vi "Winch v4.vi"() -> ()   [LabVIEW 2013]
uses:
  <vilib>/Rock Robotics/WPI/Joystick/WPI_JoystickGetSetRefNum.vi
  Robot Global Data.vi
  Globals/Useful Values.vi
  Globals/Homes.vi
  <vilib>/Utility/file.llb/Write To Spreadsheet File (DBL).vi
  <vilib>/addons/control/pid/pid.llb/PID (DBL).vi
  <vilib>/addons/control/pid/NI_PID_pid.lvlib
panel:
  in  "PID gains":T1={"proportional gain (Kc)"=2.75, "integral time (Ti, min)"=0.0, "derivative time (Td, min)"=0.0} {"derivative time (Td, min)" format="%.3f"; "integral time (Ti, min)" format="%.3f"; "proportional gain (Kc)" format="%.3f"}
  # "PULLBACK SPEED NEEDS\nTO BE NEGATIVE OR ELSE"
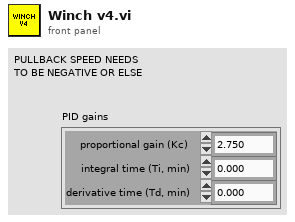
[diagram p1: front panel]
types:
  T1 = cluster{"proportional gain (Kc)":dbl, "integral time (Ti, min)":dbl, "derivative time (Td, min)":dbl}
  T2 = typedef "WPI_DigitalInputDevRef.ctl" = cluster{"DevStatus":errorcluster, "DIO Channel":T3, "Digital Module":T4}
  T3 = typedef "FPGA_DIOChannel.ctl" = enum8{"DIO 1", "DIO 2", "DIO 3", "DIO 4", "DIO 5", "DIO 6", "DIO 7", "DIO 8", "DIO 9", "DIO 10", "DIO 11", "DIO 12", "DIO 13", "DIO 14", "Invalid"}
  T4 = typedef "FPGA_TypedefDigitalModule.ctl" = enum16{"Digital Module 1", "Digital Module 2"}
  T5 = typedef "WPI_MotorControlDeviceRef.ctl" = cluster{"DeviceStatus":errorcluster, "Type":enum16{"PWM", "CAN"}, "PWM":cluster{"Digital Module":T4, "PWM Channel":T6, "DeadBand":T7}, "CAN":cluster{"Device Number":u8, "Control Mode":T8, "Semaphore":T9, "Max Vout":dbl}, "Invert":bool, "TransformRef":T10, "InvTransformRef":T10}
  T6 = typedef "FPGA_DIOPWMChannel.ctl" = enum8{"PWM 1", "PWM 2", "PWM 3", "PWM 4", "PWM 5", "PWM 6", "PWM 7", "PWM 8", "PWM 9", "PWM 10", "Invalid"}
  T7 = typedef "WPI_PWMDeadband.ctl" = cluster{"Name":string, "maxPositivePwm":i32, "minPositivePwm":i32, "centerPwm":i32, "maxNegativePwm":i32, "minNegativePwm":i32, "angularRange":u16}
  T8 = typedef "WPI_CANJaguar_ControlMode.ctl" = enum8{"Percent VBus", "Current", "Speed", "Position", "Voltage"}
  T9 = typedef "Semaphore RefNum" = refnum<k1>
  T10 = typedef "WPI_PWMTransform_ConPane.ctl" = refnum<vi>
  T11 = typedef "WPI_AnalogChannelDevRef.ctl" = cluster{"DevStatus":errorcluster, "Analog Module":T12, "Analog Channel":T13}
  T12 = typedef "FPGA_TypedefAnalogModule.ctl" = enum16{"Analog Module 1", "Analog Module 2"}
  T13 = typedef "FPGA_AIChannel.ctl" = enum8{"AI 1", "AI 2", "AI 3", "AI 4", "AI 5", "AI 6", "AI 7", "AI 8", "Invalid"}
  T14 = typedef "WPI_JoystickDevRef.ctl" = cluster{"Device":T15}
  T15 = typedef "WPI_JoystickDeviceEnum.ctl" = enum16{"USB 1", "USB 2", "USB 3", "USB 4", "Kinect 1", "Kinect 2"}
  T16 = typedef "WPI_DriverStationRobotMode2.ctl" = enum16{"Autonomous Disabled", "Autonomous Enabled", "Teleop Disabled", "Teleop Enabled", "Timeout", "Finish", "Test Disabled", "Test Enabled"}
  T17 = typedef "WPI_JoystickButtonState.ctl" = cluster{"Button 1":bool, "Button 2":bool, "Button 3":bool, "Button 4":bool, "Button 5":bool, "Button 6":bool, "Button 7":bool, "Button 8":bool, "Button 9":bool, "Button 10":bool, "Button 11":bool, "Button 12":bool}
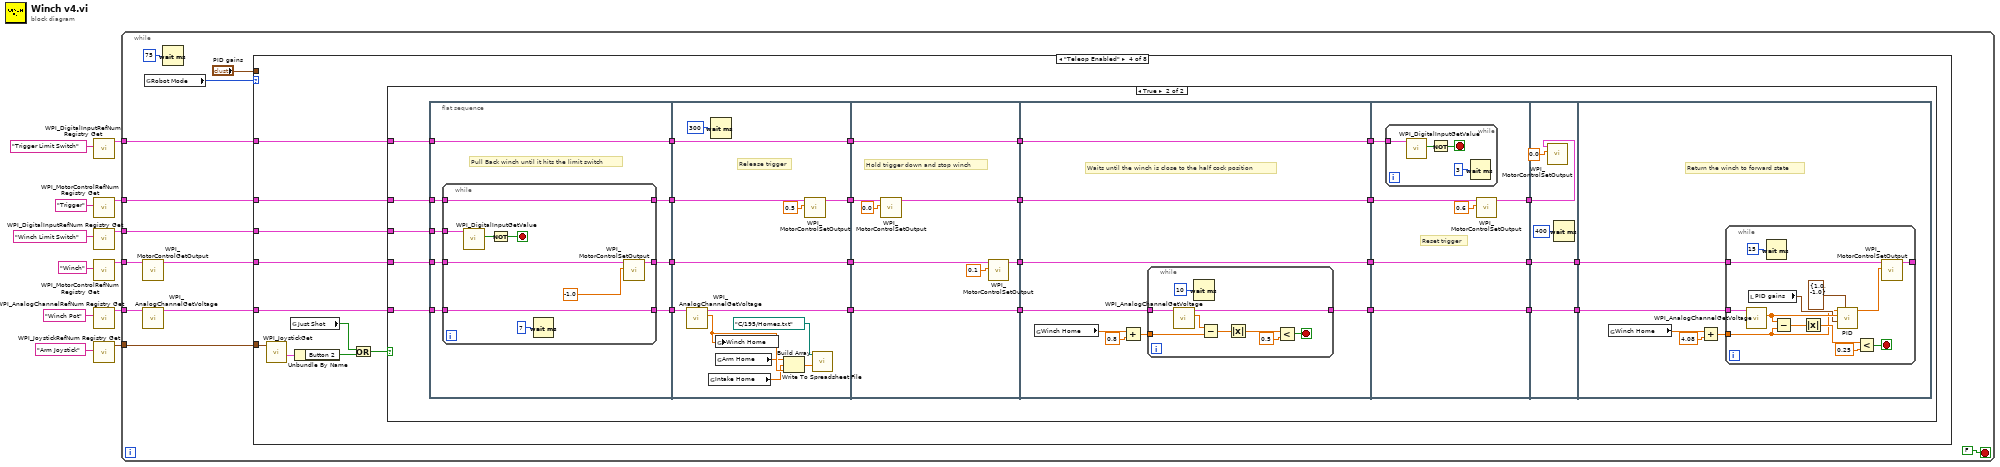
[diagram p0: block diagram]
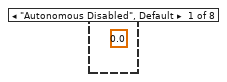
[diagram p2: hidden frame]
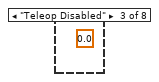
[diagram p4: hidden frame]
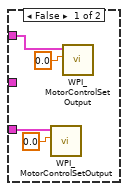
[diagram p5: hidden frame]
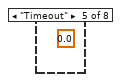
[diagram p6: hidden frame]
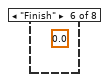
[diagram p7: hidden frame]
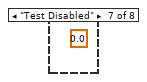
[diagram p8: hidden frame]
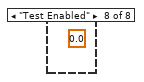
[diagram p9: hidden frame]
diagram:
  n1 = call <vilib>:"WPI_DigitalInputRefNum Registry Get.vi"("refnum name"="Trigger Limit Switch") -> ("DigitalInputDevRef"=w1:T2)  [unwired: 9 in, 1 out]
  n2 = call <vilib>:"WPI_MotorControlRefNum Registry Get.vi"("refnum name"="Trigger") -> ("MotorControlDevRef"=w3:T5)  [unwired: 9 in, 1 out]
  n3 = call <vilib>:"WPI_DigitalInputRefNum Registry Get.vi"("refnum name"="Winch Limit Switch") -> ("DigitalInputDevRef"=w6:T2)  [unwired: 9 in, 1 out]
  n4 = call <vilib>:"WPI_MotorControlRefNum Registry Get.vi"("refnum name"="Winch") -> ("MotorControlDevRef"=w9:T5)  [unwired: 9 in, 1 out]
  n5 = call <vilib>:"WPI_AnalogChannelRefNum Registry Get.vi"("refnum name"="Winch Pot") -> ("AIDeviceRef"=w12:T11)  [unwired: 9 in, 1 out]
  n6 = call <vilib>:"WPI_JoystickRefNum Registry Get.vi"("refnum name"="Arm Joystick") -> ("JoystickDevRef"=w7:T14)  [unwired: 9 in, 1 out]
  n7 = while {
    tunnel: w12 -> [w22]
    tunnel: w9 -> [w17]
    tunnel: w7 -> [w19]
    tunnel: w6 -> [w14]
    tunnel: w3 -> [w15]
    tunnel: w1 -> [w13]
    stop <- FALSE stop-if-true
    n8 = call <vilib>:"WPI_MotorControlGetOutput.vi"("MotorControlDevRef"=w17) -> ("MotorControlDevRef"=w16:T5)  [unwired: 8 in, 2 out]
    n9 = call <vilib>:"WPI_AnalogChannelGetVoltage.vi"("AIDeviceRef"=w22) -> ("AIDeviceRef"=w18:T11)  [unwired: 8 in, 2 out]
    n10 = global read "Robot Global Data.vi" "Robot Mode"() -> (w21:T16)
    n11 = Wait (ms)(milliseconds to wait=u32 75) -> ()  [unwired: 1 out]
    n12 = case shown="\"Teleop Enabled\"" w21 {
      tunnel: w16 -> [_ _ _ w31 _ _ _ _]
      tunnel: "PID gains" -> [_ _ _ _ _ _ _ _]
      tunnel: w19 -> [_ _ _ w34 _ _ _ _]
      tunnel: w14 -> [_ _ _ w32 _ _ _ _]
      tunnel: w18 -> [_ _ _ w30 _ _ _ _]
      tunnel: w15 -> [_ _ _ w26 _ _ _ _]
      tunnel: w13 -> [_ _ _ w25 _ _ _ _]
      frame "Autonomous Disabled", Default {
        (unwired) 0.0 ("Motor Output")
      }
      frame "Autonomous Enabled" {
      }
      frame "Teleop Disabled" {
        (unwired) 0.0 ("Motor Output")
      }
      frame "Teleop Enabled" {
        n13 = call <vilib>:"WPI_JoystickGet.vi"("JoystickDevRef"=w34) -> ("Buttons"=w33:T17)  [unwired: 4 in, 2 out]
        n14 = global read "Useful Values.vi" "Just Shot"() -> (w29:bool)
        n15 = Unbundle By Name(w33) -> ("Button 2"=w28:bool)
        n16 = Or(x=w29, y=w28) -> (x .or. y?=w27:bool)
        n17 = case shown="True" w27 {
          tunnel: w32 -> [_ w62]
          tunnel: w31 -> [w38 w64]
          tunnel: w30 -> [_ w63]
          tunnel: w26 -> [w35 w61]
          tunnel: w25 -> [_ w47]
          frame False {
            n18 = call <vilib>:"WPI_MotorControlSetOutput.vi"("Output"=0.0, "MotorControlDevRef"=w38) -> ()  [unwired: 7 in, 3 out]
            n19 = call <vilib>:"WPI_MotorControlSetOutput.vi"("Output"=0.0, "MotorControlDevRef"=w35) -> ()  [unwired: 7 in, 3 out]
          }
          frame True {
            n20 = flat-sequence {
              tunnel: w64 -> [w72]
              tunnel: w63 -> [w71]
              tunnel: w62 -> [w70]
              tunnel: w61 -> [w68]
              tunnel: [w69] -> w60
              tunnel: [w67] -> w57
              tunnel: [w66] -> w56
              tunnel: [w65] -> w48
              tunnel: w47 -> [w65]
              tunnel: w60 -> [w94]
              tunnel: [w91] -> w59
              tunnel: [w90] -> w58
              tunnel: w57 -> [w90]
              tunnel: w56 -> [w83]
              tunnel: [w82] -> w55
              tunnel: [w89] -> w49
              tunnel: w48 -> [w89]
              tunnel: w59 -> [w102]
              tunnel: w58 -> [w99]
              tunnel: w55 -> [w100]
              tunnel: [w100] -> w54
              tunnel: [w98] -> w53
              tunnel: [w96] -> w50
              tunnel: w49 -> [w96]
              tunnel: [w95] -> w46
              tunnel: w54 -> [w109]
              tunnel: w53 -> [w110]
              tunnel: [w110] -> w52
              tunnel: [w105] -> w51
              tunnel: w50 -> [w105]
              tunnel: w46 -> [w104]
              tunnel: [w104] -> w45
              tunnel: [w103] -> w44
              tunnel: w52 -> [w125]
              tunnel: [w125] -> w43
              tunnel: w51 -> [w124]
              tunnel: w45 -> [w122]
              tunnel: [w121] -> w41
              tunnel: w44 -> [w120]
              tunnel: [w120] -> w40
              tunnel: w43 -> [w134]
              tunnel: [w134] -> w42
              tunnel: w41 -> [w130]
              tunnel: w40 -> [w133]
              tunnel: [w133] -> w39
              tunnel: w42 -> [w139]
              tunnel: w39 -> [w138]
              frame #0 {
                # "Pull Back winch until it hits the limit switch"
                n21 = while {
                  tunnel: [w78] -> w67
                  tunnel: w72 -> [w76]
                  tunnel: w71 -> [w73]
                  tunnel: w70 -> [w75]
                  tunnel: [w74] -> w69
                  tunnel: w68 -> [w74]
                  tunnel: [w73] -> w66
                  stop <- w77 stop-if-true
                  n22 = call <vilib>:"WPI_DigitalInputGetValue.vi"("DigitalInputDevRef"=w75) -> ("Value"=w81:bool)  [unwired: 8 in, 2 out]
                  n23 = Not(x=w81) -> (.not. x?=w77:bool)
                  n24 = Wait (ms)(milliseconds to wait=u32 7) -> ()  [unwired: 1 out]
                  n25 = call <vilib>:"WPI_MotorControlSetOutput.vi"("Output"=-1.0 ("Pullback Speed"), "MotorControlDevRef"=w76) -> ("MotorControlDevRef"=w78:T5)  [unwired: 7 in, 2 out]
                }
              }
              frame #1 {
                # "Release trigger"
                n26 = call <vilib>:"WPI_AnalogChannelGetVoltage.vi"("AIDeviceRef"=w83) -> ("Voltage"=w88:dbl, "AIDeviceRef"=w82:T11)  [unwired: 8 in, 1 out]
                n27 = global read "Homes.vi" "Intake Home"() -> (w87:dbl)
                n28 = Wait (ms)(milliseconds to wait=u32 300) -> ()  [unwired: 1 out]
                n29 = global write "Homes.vi" "Winch Home"(w88) -> ()
                n30 = global read "Homes.vi" "Arm Home"() -> (w85:dbl)
                n31 = Build Array(w85, w87, w88) -> (w86:dbl[])
                n32 = call <vilib>:"WPI_MotorControlSetOutput.vi"("Output"=0.5, "MotorControlDevRef"=w94) -> ("MotorControlDevRef"=w91:T5)  [unwired: 7 in, 2 out]
                n33 = call-poly <vilib>:"Write To Spreadsheet File.vi"("1D data"=w86, "file path (dialog if empty)"=path "C:/195/Homes.txt") -> ()  [unwired: 6 in, 1 out]
              }
              frame #2 {
                # "Hold trigger down and stop winch"
                n34 = call <vilib>:"WPI_MotorControlSetOutput.vi"("Output"=0.0, "MotorControlDevRef"=w102) -> ("MotorControlDevRef"=w95:T5)  [unwired: 7 in, 2 out]
                n35 = call <vilib>:"WPI_MotorControlSetOutput.vi"("Output"=0.1, "MotorControlDevRef"=w99) -> ("MotorControlDevRef"=w98:T5)  [unwired: 7 in, 2 out]
              }
              frame #3 {
                # "Waits until the winch is close to the half cock position"
                n36 = global read "Homes.vi" "Winch Home"() -> (w108:dbl)
                n37 = Add(x=w108, y=0.8) -> (x+y=w106:dbl)
                n38 = while {
                  tunnel: w109 -> [w119]
                  tunnel: w106 -> [w112]
                  tunnel: [w111] -> w103
                  stop <- w113 stop-if-true
                  n39 = call <vilib>:"WPI_AnalogChannelGetVoltage.vi"("AIDeviceRef"=w119) -> ("Voltage"=w118:dbl, "AIDeviceRef"=w111:T11)  [unwired: 8 in, 1 out]
                  n40 = Wait (ms)(milliseconds to wait=u32 10) -> ()  [unwired: 1 out]
                  n41 = Subtract(x=w118, y=w112) -> (x-y=w117:dbl)
                  n42 = Absolute Value(x=w117) -> (abs(x)=w116:dbl)
                  n43 = Less?(x=w116, y=0.5) -> (x < y?=w113:bool)
                }
              }
              frame #4 {
                # "Reset trigger"
                n44 = while {
                  tunnel: w124 -> [w129]
                  stop <- w127 stop-if-true
                  n45 = call <vilib>:"WPI_DigitalInputGetValue.vi"("DigitalInputDevRef"=w129) -> ("Value"=w128:bool)  [unwired: 8 in, 2 out]
                  n46 = Not(x=w128) -> (.not. x?=w127:bool)
                  n47 = Wait (ms)(milliseconds to wait=u32 3) -> ()  [unwired: 1 out]
                }
                n48 = call <vilib>:"WPI_MotorControlSetOutput.vi"("Output"=0.6, "MotorControlDevRef"=w122) -> ("MotorControlDevRef"=w121:T5)  [unwired: 7 in, 2 out]
              }
              frame #5 {
                n49 = call <vilib>:"WPI_MotorControlSetOutput.vi"("Output"=0.0, "MotorControlDevRef"=w130) -> ()  [unwired: 7 in, 3 out]
                n50 = Wait (ms)(milliseconds to wait=u32 400) -> ()  [unwired: 1 out]
              }
              frame #6 {
                # "Return the winch to forward state"
                n51 = global read "Homes.vi" "Winch Home"() -> (w137:dbl)
                n52 = Add(x=w137, y=4.08) -> (x+y=w135:dbl)
                n53 = while {
                  tunnel: w139 -> [w152]
                  tunnel: [w145] -> _
                  tunnel: w138 -> [w141]
                  tunnel: w135 -> [w140]
                  stop <- w149 stop-if-true
                  n54 = call <vilib>:"WPI_AnalogChannelGetVoltage.vi"("AIDeviceRef"=w141) -> ("Voltage"=w146:dbl)  [unwired: 8 in, 2 out]
                  n55 = local read "PID gains"() -> (w144:T1)
                  n56 = Wait (ms)(milliseconds to wait=u32 15) -> ()  [unwired: 1 out]
                  n57 = Subtract(x=w146, y=w140) -> (x-y=w151:dbl)
                  n58 = Absolute Value(x=w151) -> (abs(x)=w150:dbl)
                  n59 = call-poly <vilib>:"PID.vi"("output range"=cluster{"output high":dbl, "output low":dbl} {"output high"=1.0, "output low"=-1.0}, "PID gains"=w144, "process variable"=w146, "setpoint"=w140) -> ("output"=w142:dbl)  [unwired: 6 in, 1 out]
                  n60 = Less?(x=w150, y=0.25) -> (x < y?=w149:bool)
                  n61 = call <vilib>:"WPI_MotorControlSetOutput.vi"("Output"=w142, "MotorControlDevRef"=w152) -> ("MotorControlDevRef"=w145:T5)  [unwired: 7 in, 2 out]
                }
              }
            }
          }
        }
      }
      frame "Timeout" {
        (unwired) 0.0 ("Motor Output")
      }
      frame "Finish" {
        (unwired) 0.0 ("Motor Output")
      }
      frame "Test Disabled" {
        (unwired) 0.0 ("Motor Output")
      }
      frame "Test Enabled" {
        (unwired) 0.0 ("Motor Output")
      }
    }
  }
